vi "HumanGlobal.vi"() -> ()   [LabVIEW 2023]
uses:
  HumanDriveModeENUM.ctl
panel:
  out "Human_DebugButtonRecv":bool
  out "TrajDesiredOrientation_Deg":dbl
  out "TrajDesiredY_Ft":dbl=13.0
  out "TrajDesiredX_Ft":dbl=10.0
  out "Human_DriveFIeldOriented":bool
  out "Human_DriveMode":T1
  # "DESIRED ABS POSE FOR TRAJECTORY"
  # "DRIVING MODES"
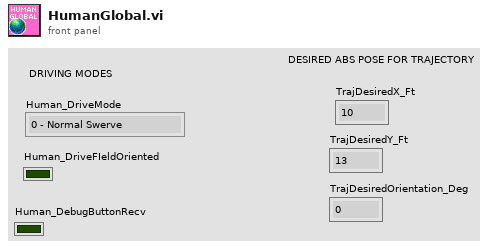
[diagram p1: front panel]
types:
  T1 = typedef "HumanDriveModeENUM.ctl" = enum16{"0 - Normal Swerve", "1 - Auto traj  - Left Speaker", "2 - Auto traj - Center Speaker", "3 - Auto traj - Speaker Right", "4 - Auto traj - Amp", "5 - Auto traj - Source", "6 - Auto traj -  Left Stage", "7 - Auto traj - Center Stage", "8 - Auto traj - Right Stage"}
diagram:
